vi "Build Array Function.vi"() -> ()   [LabVIEW 2012]
panel:
  out "2-D Array":i32[][](array[numeric])
  out "Concatenated Array":i32[](array[numeric])
  out "Appended Element":i32[](array[numeric])
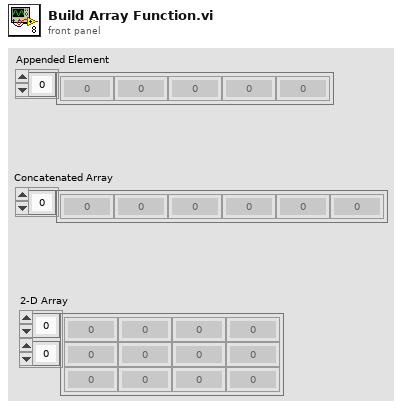
[diagram p1: front panel]
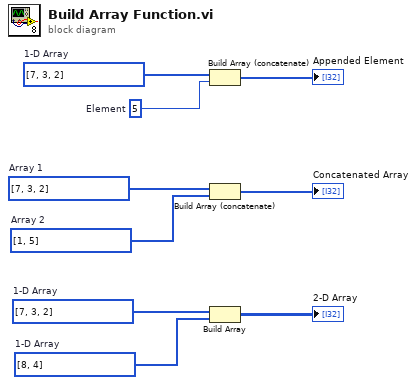
[diagram p0: block diagram]
diagram:
  w3 = i32[] [8, 4]  # 1-D Array
  w2 = i32[] [7, 3, 2]  # 1-D Array
  w4 = i32[] [1, 5]  # Array 2
  w5 = i32[] [7, 3, 2]  # Array 1
  w8 = 5  # Element
  w9 = i32[] [7, 3, 2]  # 1-D Array
  n1 = Build Array (concatenate) "Build Array"(w9, w8) -> (→"Appended Element":i32[])
  n2 = Build Array (concatenate) "Build Array"(w5, w4) -> (→"Concatenated Array":i32[])
  n3 = Build Array "Build Array"(w2, w3) -> (→"2-D Array":i32[][])
